vi "强制手动.vi"(8 "error in (no error)":errorcluster, 11 "强制手动":bool) -> (0 "error out":errorcluster)   [LabVIEW 2016, in "PLC.lvlib"]
uses:
  PLC.lvlib
  <vilib>/Plasmionique/MB Master/MB_Master_Serial/MB_Master_Serial.lvclass
  C:/Program Files (x86)/National Instruments/LabVIEW 2016/vi.lib/Plasmionique/MB Master/MB_Master/MB_Master.lvclass
  <vilib>/Plasmionique/MB Master/MB Master.lvlib
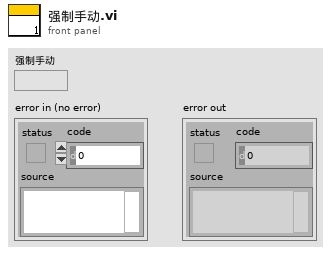
[diagram p1: front panel]
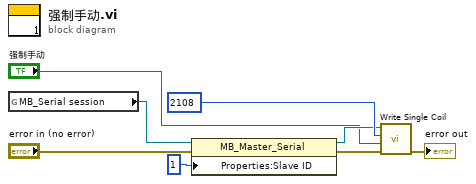
[diagram p0: block diagram]
diagram:
  n1 = global read "中间变量.vi" "MB_Serial session"() -> (w6:refnum<class "MB_Master_Serial.lvclass">)
  n2 = property class="MB_Master_Serial"(reference=w6, error in="error in (no error)", "Properties:Slave ID"=u8 1 ("Slave ID")) -> (reference out=w5:refnum<class "MB_Master_Serial.lvclass">, error out=w2:errorcluster)
  n3 = call <vilib>:"Write Single Coil.vi"("error in (no error)"=w2, "value"="强制手动", "address"=2108, "MB session in"=w5) -> ("error out"=→"error out":errorcluster)  [unwired: 6 in, 1 out]
